vi "父项目与子项目.vi"() -> ()   [LabVIEW 2012, in "Tree Tools.lvlib"]
uses:
  Tree Tools.lvlib
  Core Class/Tree Class/Tree Class.lvclass
  Core Class/Tree Tag Class/Tree Tag Class.lvclass
panel:
  out "Children Tag Strings":string[](array[string])
  out "Parent Tag string":string
  in  "停止":bool
  in  "树形":string(tree)
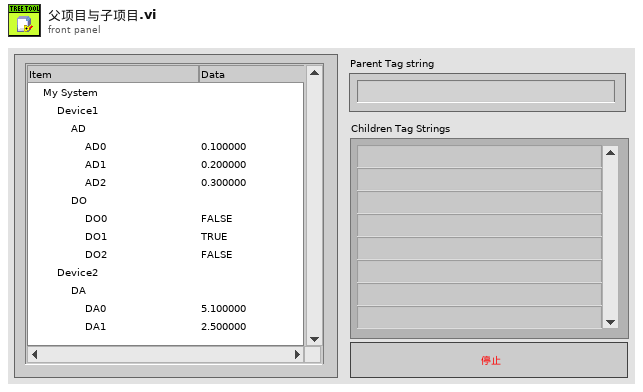
[diagram p1: front panel]
types:
  T1 = cluster{"Device1":cluster{"AD":cluster{"AD0":dbl, "AD1":dbl, "AD2":dbl}, "DO":cluster{"DO0":bool, "DO1":bool, "DO2":bool}}, "Device2":cluster{"DA":cluster{"DA0":dbl, "DA1":dbl, "DA2":dbl}, "DI":cluster{"DI0":bool, "DI1":bool, "DI2":bool}}}
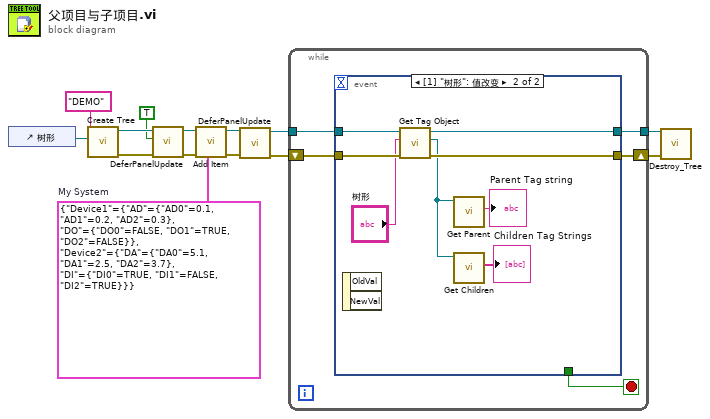
[diagram p0: block diagram]
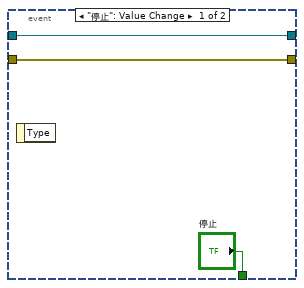
[diagram p2: hidden frame]
diagram:
  w7 = T1 {"Device1"={"AD"={"AD0"=0.1, "AD1"=0.2, "AD2"=0.3}, "DO"={"DO0"=FALSE, "DO1"=TRUE, "DO2"=FALSE}}, "Device2"={"DA"={"DA0"=5.1, "DA1"=2.5, "DA2"=3.7}, "DI"={"DI0"=TRUE, "DI1"=FALSE, "DI2"=TRUE}}}  # My System
  n1 = control-ref of="树形"() -> (w14:refnum<vi>)
  n2 = call "Create Tree.vi"("Tree Refnum"=w14, "Tree Name"="DEMO") -> ("error out"=w11:errorcluster, "Tree_LVOOP out"=w12:refnum<class "Tree Class.lvclass">)  [unwired: 8 in]
  n3 = call-dynamic "DeferPanelUpdate.vi"("error in (no error)"=w11, "Defer? (F)"=TRUE, "Tree_LVOOP__lava_lib_tree_class in"=w12) -> ("error out"=w8:errorcluster, "Tree_LVOOP__lava_lib_tree_class out"=w9:refnum<class "Tree Class.lvclass">)  [unwired: 7 in]
  n4 = call-dynamic "Add Item.vi"("Data"=w7, "error in (no error)"=w8, "Tree_LVOOP in"=w9) -> ("error out"=w5:errorcluster, "Tree_LVOOP out"=w6:refnum<class "Tree Class.lvclass">)  [unwired: 6 in, 1 out]
  n5 = call-dynamic "DeferPanelUpdate.vi"("error in (no error)"=w5, "Tree_LVOOP__lava_lib_tree_class in"=w6) -> ("error out"=w4:errorcluster, "Tree_LVOOP__lava_lib_tree_class out"=w3:refnum<class "Tree Class.lvclass">)  [unwired: 8 in]
  n6 = while {
    shift-right: [w16] -> w1
    shift-left: w4 -> [w17]
    tunnel: w3 -> [w18]
    tunnel: [w15] -> w2
    stop <- w19 stop-if-true
    n7 = event shown="[1] \"树形\": 值改变" {
      selector: _ -> [_ _]
      dyn-events: _ -> [_ _]
      timeout: _ -> [_ _]
      tunnel: ["停止" _] -> w19
      tunnel: w18 -> [w21 w30]
      tunnel: w17 -> [w20 w29]
      tunnel: [w21 w27] -> w15
      tunnel: [w20 w26] -> w16
      event "停止": Value Change {
        n8 = event-data() -> ()  [unwired: 1 in, 1 out]
      }
      event "树形": Value Change {
        n9 = event-data() -> ()  [unwired: 1 in, 2 out]
        n10 = call-dynamic "Get Tag Object.vi"("error in (no error)"=w29, "Tag (string)"="树形", "Tree_LVOOP in"=w30) -> ("error out"=w26:errorcluster, "Tag"=w25:refnum<class "Tree Tag Class.lvclass">, "Tree_LVOOP out"=w27:refnum<class "Tree Class.lvclass">)  [unwired: 5 in, 1 out]
        n11 = call-dynamic "Get Parent.vi"("Tag_LVOOP in"=w25) -> ("Parent Tag string"=→"Parent Tag string":string)  [unwired: 7 in, 3 out]
        n12 = call-dynamic "Get Children.vi"("Tag_LVOOP in"=w25) -> ("Children Tag Strings"=→"Children Tag Strings":string[])  [unwired: 7 in, 3 out]
      }
    }
  }
  n13 = call-dynamic "Destroy_Tree.vi"("error in (no error)"=w1, "Tree_LVOOP in"=w2) -> ()  [unwired: 9 in, 1 out]
